vi "Examen.vi"() -> ()   [LabVIEW 2020]
panel:
  out "Lim max":dbl=60.0
  in  "stop":bool
  out "Rango":bool
  out "Histeresis":bool
  in  "Min":dbl=38.0
  in  "Max":dbl=60.0
  out "Numero Aleatorio":dbl
  out "Waveform Chart":cluster{dbl, dbl}(graph)={115.7263656527014, 70.2583861115194}
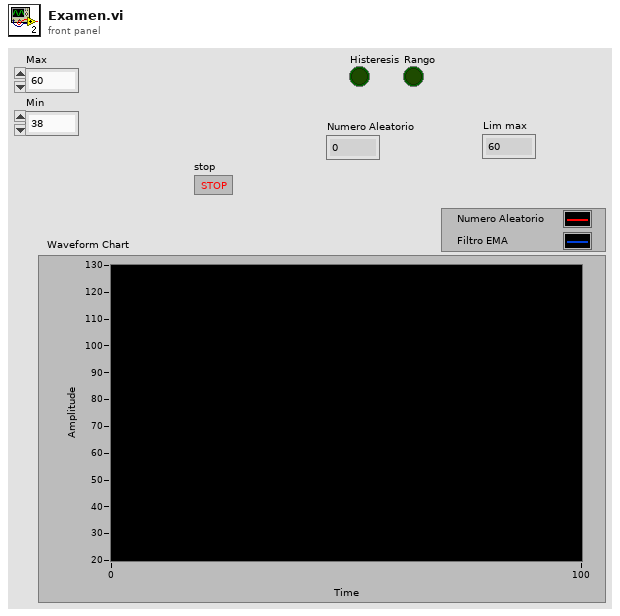
[diagram p1: front panel]
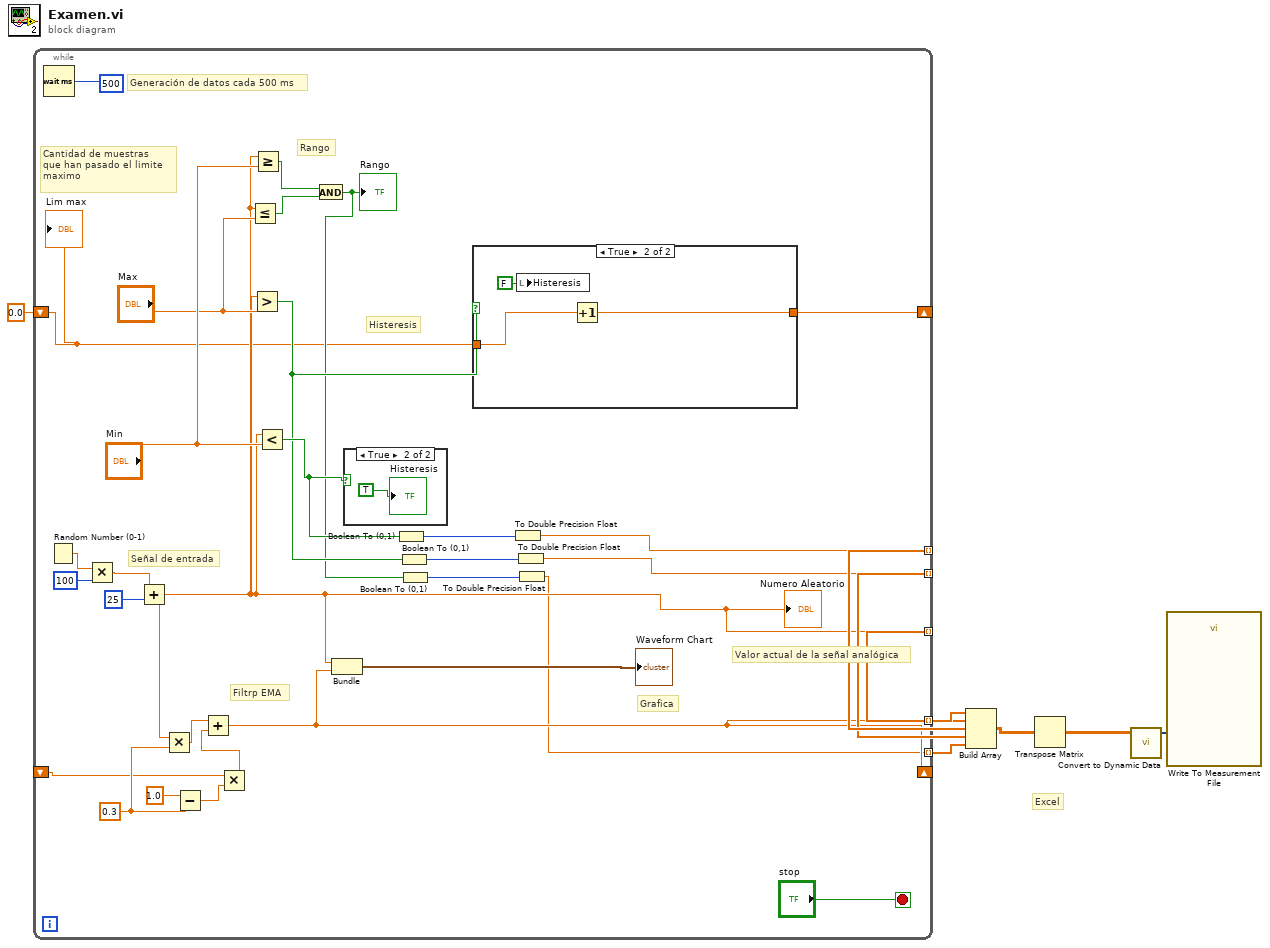
[diagram p0: block diagram]
diagram:
  # "Excel"
  n1 = while {
    shift-right: [w24] -> _
    shift-left: _ -> [w35]
    tunnel: [w24] -> w6 mode=indexing
    tunnel: [w23] -> w5 mode=indexing
    tunnel: [w19] -> w4 mode=indexing
    tunnel: [w16] -> w3 mode=indexing
    tunnel: [w13] -> w2 mode=indexing
    shift-right: [w11] -> _
    shift-left: 0.0 -> [w10]
    stop <- "stop" stop-if-true
    w36 = 0.3 ("y")
    # "Generación de datos cada 500 ms"
    # "Cantidad de muestras \nque han pasado el limite \nmaximo"
    # "Valor actual de la señal analógica"
    # "Grafica"
    # "Rango"
    # "Histeresis"
    # "Señal de entrada"
    # "Filtrp EMA"
    n2 = Wait (ms)(milliseconds to wait=u32 500) -> ()  [unwired: 1 out]
    n3 = Random Number (0-1)() -> (number: 0 to 1=w27:dbl)
    n4 = Multiply(x=w27, y=100) -> (x*y=w25:dbl)
    n5 = Add(x=w25, y=25) -> (x+y=w23:dbl)
    "Numero Aleatorio" <- w23
    n6 = Multiply(x=w23, y=w36) -> (x*y=w34:dbl)
    n7 = Subtract(x=1.0, y=w36) -> (x-y=w38:dbl)
    n8 = Multiply(x=w35, y=w38) -> (x*y=w33:dbl)
    n9 = Add(x=w34, y=w33) -> (x+y=w24:dbl)
    n10 = Less Or Equal?(x=w23, y="Max") -> (x <= y?=w31:bool)
    n11 = Greater?(x=w23, y="Max") -> (0:w17:bool)
    n12 = Greater Or Equal?(x=w23, y="Min") -> (x >= y?=w32:bool)
    n13 = Less?(x=w23, y="Min") -> (x < y?=w22:bool)
    n14 = And(x=w32, y=w31) -> (x .and. y?=w14:bool)
    "Rango" <- w14
    n15 = Bundle(w23, w24) -> (→"Waveform Chart":cluster{dbl, dbl})  [unwired: 1 in]
    n16 = case shown="True" w22 {
      frame False {
      }
      frame True {
        "Histeresis" <- TRUE
      }
    }
    n17 = Boolean To (0,1)(Boolean=w22) -> (0, 1=w20:i16)
    n18 = Boolean To (0,1)(Boolean=w17) -> (0, 1=w18:i16)
    n19 = Boolean To (0,1)(Boolean=w14) -> (0, 1=w15:i16)
    n20 = case shown="True" w17 {
      tunnel: [w41 w43] -> w11
      tunnel: w10 -> [w41 w42]
      frame False {
      }
      frame True {
        n21 = local write "Histeresis"(FALSE) -> ()
        n22 = Increment(x=w42) -> (x+1=w43:dbl)
      }
    }
    n23 = To Double Precision Float(number=w20) -> (double precision float=w19:dbl)
    n24 = To Double Precision Float(number=w18) -> (double precision float=w16:dbl)
    n25 = To Double Precision Float(number=w15) -> (double precision float=w13:dbl)
    "Lim max" <- w10
  }
  n26 = Build Array(w6, w5, w4, w3, w2) -> (w7:dbl[][])
  n27 = Transpose Matrix(1:w7) -> (0:w9:dbl[][])
  n28 = call "Convert to Dynamic Data"("2D Array"=w9) -> ("Dynamic Data Type"=w8:dynamicdata)  [unwired: 3 in]
  n29 = call "Write To Measurement File"("Signals"=w8) -> ()  [unwired: 16 in, 3 out]
